vi "Clone VIs FG.vi"(7 "Action":T1, 8 "error in":errorcluster) -> (0 "error out":errorcluster, 3 "VIs":string[](array[string]))   [LabVIEW 2013, in "LVTM.lvlib"]
doc: "Drop this VI into any asynchronously called reentrant VI, to force it to be seen by LabVIEW Task Manager. There is no need to drop this into a statically called reentrant VI, because these are already searched for by the tool. When the reentrant clone is created and run, it will add its name to this Functional Global. LabVIEW Task Manager will now display \"All VIs in Memory\" AND the ones in this FG. Leaving this FG in your VI, even when deploying your application, will not effect the performance as it is merely an array of a few strings."
uses:
  LVTM.lvlib
  Clone VIs FG Enum.ctl
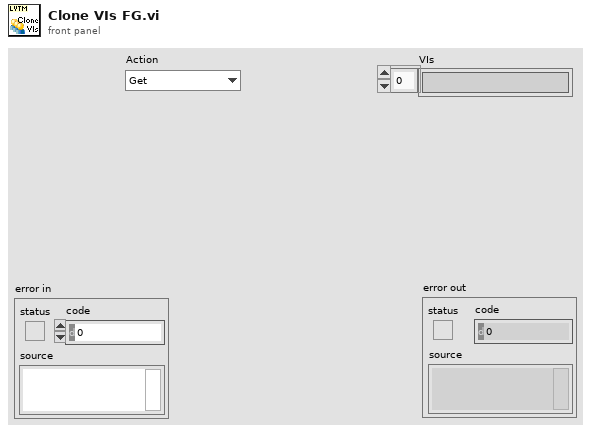
[diagram p1: front panel]
types:
  T1 = typedef "LVTM.lvlib/Clone VIs FG Enum.ctl" = enum16{"Get", "Get Active VIs", "Add Calling VI"}
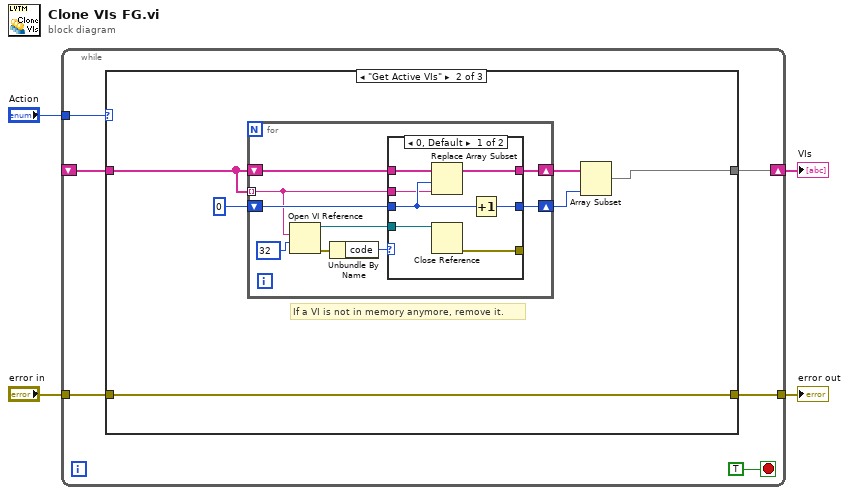
[diagram p0: block diagram]
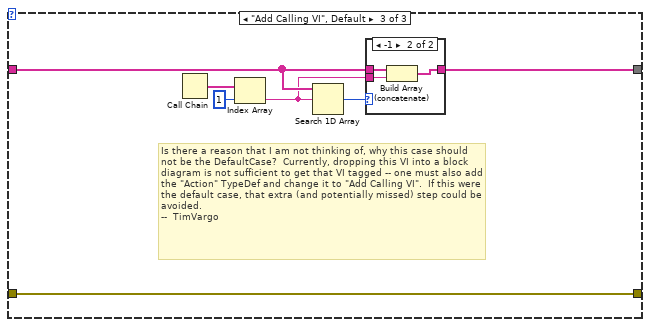
[diagram p4: hidden frame]
diagram:
  n1 = while {
    tunnel: "Action" -> [w9]
    shift-right: [w8] -> w1
    shift-left: _ -> [w7]
    tunnel: "error in" -> [w6]
    tunnel: [w5] -> w2
    stop <- TRUE stop-if-true
    n2 = case shown="\"Get Active VIs\"" w9 {
      tunnel: [w11 w13 w41] -> w8
      tunnel: w7 -> [w11 w14 w42]
      tunnel: w6 -> [w12 w18 w43]
      tunnel: [w12 w18 w43] -> w5
      frame "Get" {
      }
      frame "Get Active VIs" {
        # "If a VI is not in memory anymore, remove it."
        n3 = for {
          shift-right: [w23] -> w16
          shift-left: w14 -> [w24]
          tunnel: w14 -> [w20] mode=indexing
          shift-right: [w22] -> w15
          shift-left: 0 -> [w21]
          n4 = Open VI Reference(vi path=w20, options=32) -> (vi reference=w25:refnum<vi>, error out=w27:errorcluster)  [unwired: 4 in]
          n5 = Unbundle By Name(w27) -> ("code"=w26:i32)
          n6 = case shown="0, Default" w26 {
            tunnel: w25 -> [w34 _]
            tunnel: w24 -> [w33 w36]
            tunnel: [w30 w36] -> w23
            tunnel: [w31 w35] -> w22
            tunnel: w21 -> [w32 w35]
            tunnel: [w29 _] -> _
            tunnel: w20 -> [w28 _]
            frame 0, Default {
              n7 = Replace Array Subset(array=w33, new element=w28, index=w32) -> (w30:string[])
              n8 = Close Reference(reference=w34) -> (error out=w29:errorcluster)  [unwired: 1 in]
              n9 = Increment(x=w32) -> (x+1=w31:i32)
            }
            frame 1004 {
              # "VI is not in memory"
            }
          }
        }
        n10 = Array Subset(array=w16, length=w15) -> (w13:string[])  [unwired: 1 in]
      }
      frame "Add Calling VI", Default {
        # "Is there a reason that I am not thinking of, why this case should not be the DefaultCase?  Currently, dropping this VI into a block diagram is not sufficient to get that VI tagged -- one must also add the \"Action\" TypeDef and change it to \"Add Calling VI\".  If this were the default case, that extra (and potentially missed) step could be avoided.\n--  TimVargo"
        n11 = Call Chain() -> (call chain=w40:string[])
        n12 = Index Array(array=w40, index=1) -> (element=w38:string)
        n13 = Search 1D Array(1D array=w42, element=w38) -> (index of element=w37:i32)  [unwired: 1 in]
        n14 = case shown="-1" w37 {
          tunnel: w42 -> [w44 w47]
          tunnel: [w44 w46] -> w41
          tunnel: w38 -> [_ w45]
          frame 0, Default {
          }
          frame -1 {
            n15 = Build Array (concatenate)(w47, w45) -> (w46:string[])
          }
        }
      }
    }
  }
  "error out" <- w2
  "VIs" <- w1
